vi "Change Delay Method.vi"(8 "error in (no error)":errorcluster, 10 "Is absolute delay mode?":bool, 11 "User Interface in":refnum<class "User Interface.lvclass">) -> (0 "error out":errorcluster, 3 "User Interface out":refnum<class "User Interface.lvclass">)   [LabVIEW 2016, in "User Interface.lvlib" / "User Interface.lvclass"]
uses:
  User Interface.lvclass
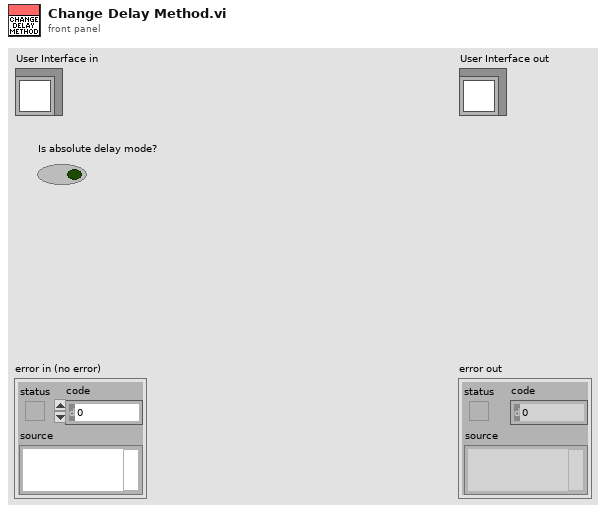
[diagram p1: front panel]
types:
  T1 = enum8{"Enabled", "Disabled", "Disabled and Grayed Out"}
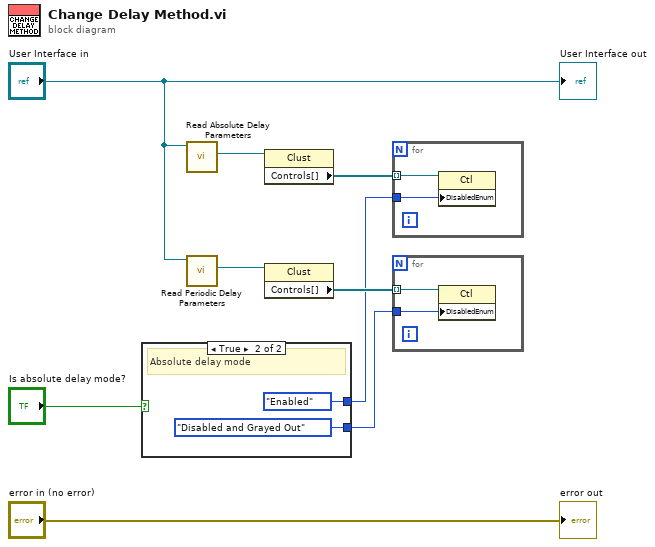
[diagram p0: block diagram]
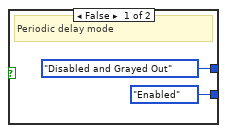
[diagram p2: hidden frame]
diagram:
  n1 = case shown="True" "Is absolute delay mode?" {
    tunnel: [T1."Disabled and Grayed Out" ("Disabled") T1."Enabled" ("Disabled")] -> w4
    tunnel: [T1."Enabled" ("Disabled") T1."Disabled and Grayed Out" ("Disabled")] -> w3
    frame False {
      # "Periodic delay mode"
    }
    frame True {
      # "Absolute delay mode"
    }
  }
  n2 = call-dynamic "Read Absolute Delay Parameters.vi"("User Interface in"="User Interface in") -> ("Absolute Delay Parameters"=w9:refnum<vi>)  [unwired: 9 in, 1 out]
  n3 = call-dynamic "Read Periodic Delay Parameters.vi"("User Interface in"="User Interface in") -> ("Periodic Delay Parameters"=w8:refnum<vi>)  [unwired: 9 in, 1 out]
  n4 = property class="Clust"(reference=w9) -> ("Controls[]"=w7:refnum<vi>[])  [unwired: 1 in, 2 out]
  n5 = property class="Clust"(reference=w8) -> ("Controls[]"=w6:refnum<vi>[])  [unwired: 1 in, 2 out]
  n6 = for {
    tunnel: w7 -> [w15] mode=indexing
    tunnel: w4 -> [w14]
    n7 = property class="Ctl"(reference=w15, "DisabledEnum"=w14) -> ()  [unwired: 1 in, 2 out]
  }
  n8 = for {
    tunnel: w6 -> [w17] mode=indexing
    tunnel: w3 -> [w16]
    n9 = property class="Ctl"(reference=w17, "DisabledEnum"=w16) -> ()  [unwired: 1 in, 2 out]
  }
  "error out" <- "error in (no error)"
  "User Interface out" <- "User Interface in"
